vi "CE14_Globals.vi"() -> ()   [LabVIEW 2018]
panel:
  in  "Read kvar":string="\u0001R1\u00021.0.3.7.0()\u0003V"
  in  "Read kW":string="\u0001R1\u00021.0.1.7.0()\u0003T"
  in  "Read Frequency":string="\u0001R1\u00021.0.14.7.0()\u0003`"
  in  "Read Power Factor":string="\u0001R1\u00021.0.13.7.0()\u0003g"
  in  "Read Voltage":string="\u0001R1\u00021.0.12.7.0()\u0003f"
  in  "Read Current":string="\u0001R1\u00021.0.11.7.0()\u0003e"
  in  "Close Connection":string="\u0001B0\u0003q"
  in  "Init4(4800)":string="\u0001P1\u0002(00000000)\u0003a"
  in  "Init3(4800)":string="\u0001P0\u0002(GELEX)\u00033"
  in  "Init2(300)":string="\u000604\r\n"
  in  "Init1(300)":string="/?!\r\n"
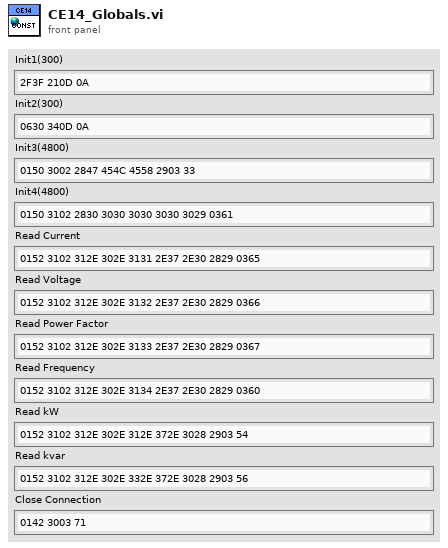
[diagram p1: front panel]
diagram:
